vi "mxwScript_Cmnd2Str_uniquifyObjects.vi"(8 "error in (no error)":errorcluster, 11 "data":variant) -> (0 "error out":errorcluster, 3 "outputString":string)   [LabVIEW 2020]
uses:
  codeGenAPISupport.llb/cgAPI_mxwScript_Unq_UniquificationData.ctl
  codeGenAPISupport.llb/cgAPI_mxwScript_uniquificationLevel.ctl
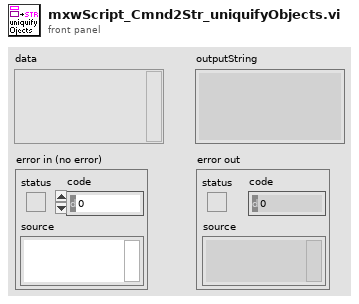
[diagram p1: front panel]
types:
  T1 = typedef "cgAPI_mxwScript_Unq_UniquificationData.ctl" = cluster{"template index":i32, "uniqificationLevel":T2}
  T2 = typedef "cgAPI_mxwScript_uniquificationLevel.ctl" = enum16{"all", "root"}
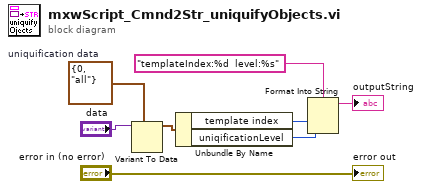
[diagram p0: block diagram]
diagram:
  w6 = T1 {"template index"=0, "uniqificationLevel"=enum."all"}  # uniquification data
  n1 = Variant To Data(type=w6, Variant="data") -> (data=w5:T1)  [unwired: 1 in, 1 out]
  n2 = Unbundle By Name(w5) -> ("template index"=w3:i32, "uniqificationLevel"=w2:T2)
  n3 = Format Into String(format string="templateIndex:%d  level:%s", w3, w2) -> (resulting string=→"outputString":string)  [unwired: 2 in, 1 out]
  "error out" <- "error in (no error)"
